vi "fetchFromTarget.vi"(8 "error in (no error)":errorcluster, 10 "ConnectionData":T1, 11 "ConfigXMLControls":T2) -> (0 "error out":errorcluster, 1 "nameMessageOut":string, 2 "SuccessfulRead?":bool, 3 "path out":path, 4 "NameTagFound":bool)   [LabVIEW 2015]
uses:
  ConfigXMLControl.ctl
  General/CorePluginInfo.ctl
  General/RemoteFiles/connectionData.ctl
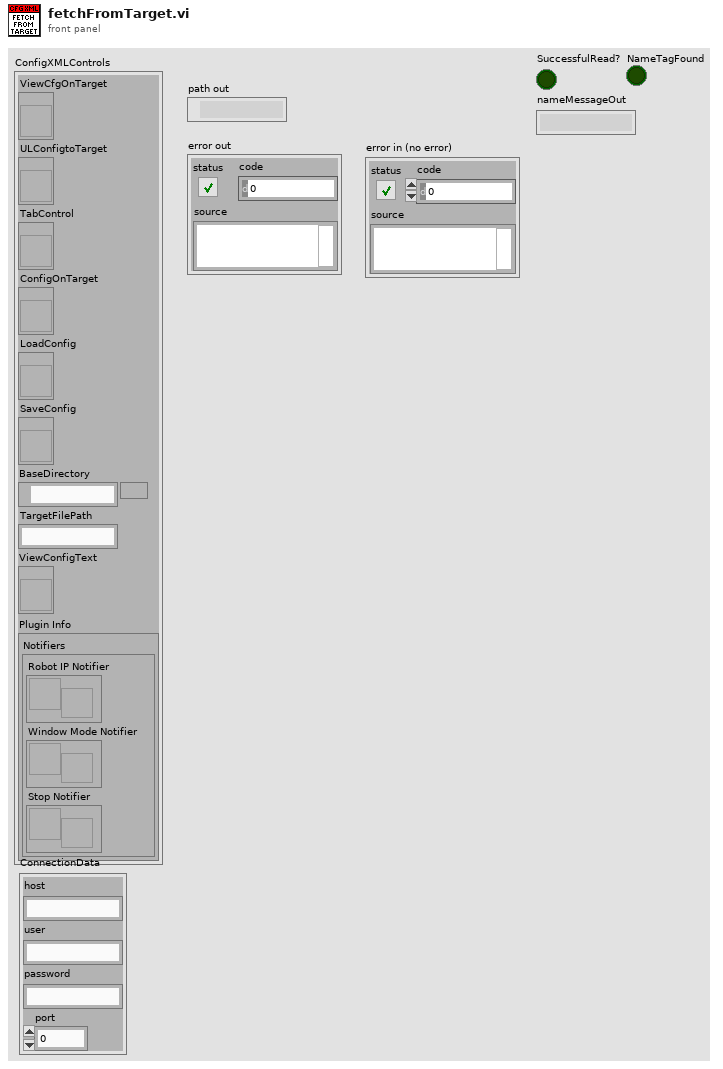
[diagram p1: front panel]
types:
  T1 = typedef "connectionData.ctl" = cluster{"host":string, "user":string, "password":string, "port":u16}
  T2 = typedef "ConfigXMLControl.ctl" = cluster{"ViewCfgOnTarget":refnum<vi>, "ULConfigtoTarget":refnum<vi>, "TabControl":refnum<vi>, "ConfigOnTarget":refnum<vi>, "LoadConfig":refnum<vi>, "SaveConfig":refnum<vi>, "BaseDirectory":path, "TargetFilePath":string, "ViewConfigText":refnum<vi>, "Plugin Info":T3}
  T3 = typedef "CorePluginInfo.ctl" = cluster{"Notifiers":cluster{"Robot IP Notifier":refnum<notifier>, "Window Mode Notifier":refnum<notifier>, "Stop Notifier":refnum<notifier>}}
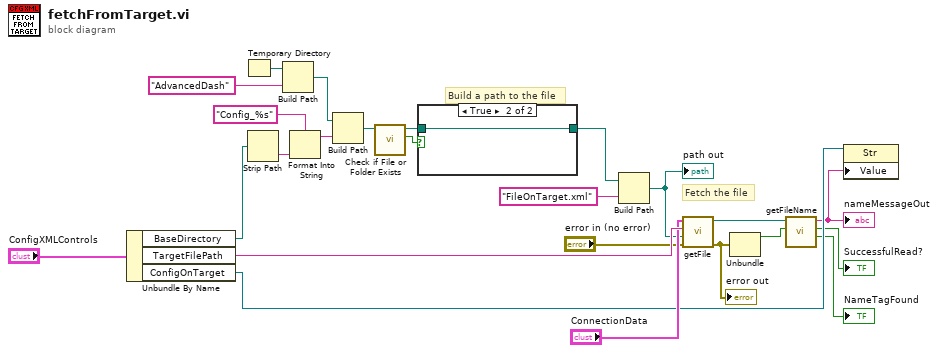
[diagram p0: block diagram]
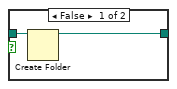
[diagram p2: hidden frame]
diagram:
  # "Build a path to the file"
  # "Fetch the file"
  n1 = Unbundle By Name("ConfigXMLControls") -> ("BaseDirectory"=w12:path, "TargetFilePath"=w24:string, "ConfigOnTarget"=w5:refnum<vi>)
  n2 = Temporary Directory() -> (w13:path)
  n3 = Strip Path(path=w12) -> (name=w18:string)  [unwired: 1 out]
  n4 = Build Path(base path=w13, name or relative path="AdvancedDash") -> (appended path=w15:path)
  n5 = Format Into String(format string="Config_%s", w18) -> (resulting string=w16:string)  [unwired: 2 in, 1 out]
  n6 = Build Path(base path=w15, name or relative path=w16) -> (appended path=w19:path)
  n7 = call <vilib>:"Check if File or Folder Exists.vi"("path"=w19) -> ("file or folder exists?"=w20:bool, "dup path"=w21:path)  [unwired: 8 in, 1 out]
  n8 = case shown="True" w20 {
    tunnel: w21 -> [w26 w27]
    tunnel: [w25 w27] -> w22
    frame False {
      n9 = Create Folder(path (use dialog)=w26) -> (created path=w25:path)  [unwired: 2 in, 2 out]
    }
    frame True {
    }
  }
  n10 = Build Path(base path=w22, name or relative path="FileOnTarget.xml") -> (appended path=w9:path)
  "path out" <- w9
  n11 = call "getFile.vi"("error in (no error)"="error in (no error)", "local path"=w9, "remote path"=w24, "ConnectionData"="ConnectionData") -> ("error out"=w6:errorcluster, "local path out"=w7:path)  [unwired: 6 in]
  "error out" <- w6
  n12 = Unbundle(w6) -> ("status"=w8:bool)  [unwired: 2 out]
  n13 = call "getFileName.vi"("File not found?"=w8, "Path"=w7) -> ("NameTagFound"=→"NameTagFound":bool, "SuccessfulRead?"=→"SuccessfulRead?":bool, "Filename"=w4:string)  [unwired: 7 in]
  "nameMessageOut" <- w4
  n14 = property class="Str"(reference=w5, "Value"=w4) -> ()  [unwired: 1 in, 2 out]
